vi "Parallel Executing Test Code.vi"(9 "Test Complete Event":refnum<user-event>, 10 "Positions":u32[](array[numeric]), 11 "Parallel Test in":refnum<class "Parallel Test.lvclass">) -> ()   [LabVIEW 2015, in "Parallel Test.lvclass"]
uses:
  Parallel Test.lvclass
  typedefs/Parallel Return -- Cluster.ctl
  Parallel Test.lvclass/Parallel Test.ctl
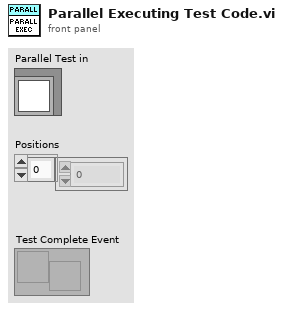
[diagram p1: front panel]
types:
  T1 = typedef "Parallel Test.lvclass/Parallel Return -- Cluster.ctl" = cluster{"Status":bool[], "Code":i32, "Source":string, "Position":u32[]}
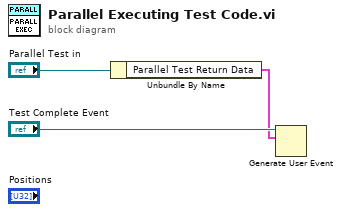
[diagram p0: block diagram]
diagram:
  n1 = Unbundle By Name("Parallel Test in") -> ("Parallel Test Return Data"=w1:T1)
  n2 = Generate User Event(user event="Test Complete Event", event data cluster=w1) -> ()  [unwired: 2 in, 2 out]
